vi "签名.vi"(10 "consumer secret":string, 11 "Signature Base string":string) -> (3 "Encoded Signature":string)   [LabVIEW 2016]
uses:
  <vilib>/LVH/i3 OAuth/Controls/Signature Method.ctl
  <vilib>/LVH/i3 External Encryption/labviewencryption/hash-types.ctl
  <vilib>/LVH/i3 External Encryption/i3-external-encryption.lvlib
  <vilib>/LVH/i3 OAuth/i3-oauth.lvlib
panel:
  out "长度":i32
  out "Base64 String":string
  in  "Signature Method":T1=enum."HMAC-SHA1"
  out "error out":errorcluster
  in  "error in (no error)":errorcluster
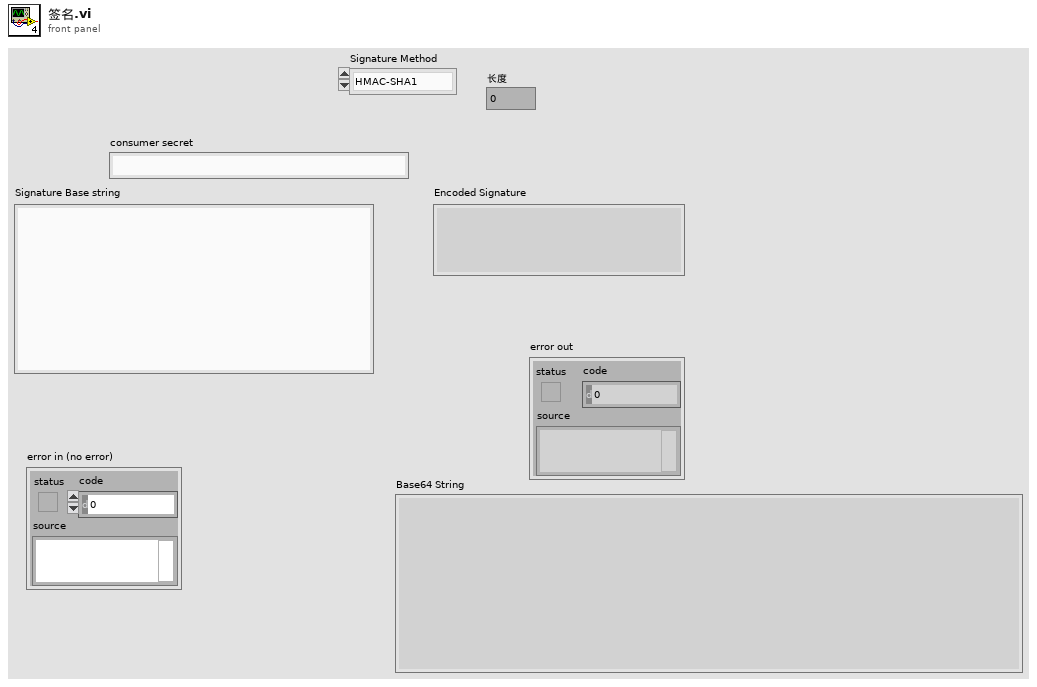
[diagram p1: front panel]
types:
  T1 = typedef "i3-oauth.lvlib/Signature Method.ctl" = enum16{"HMAC-MD5", "HMAC-SHA1", "HMAC-SHA224", "HMAC-SHA256", "HMAC-SHA384", "HMAC-SHA512"}
  T2 = typedef "i3-external-encryption.lvlib/hash-types.ctl" = enum16{"MD5", "SHA-1", "SHA-224", "SHA-256", "SHA-384", "SHA-512"}
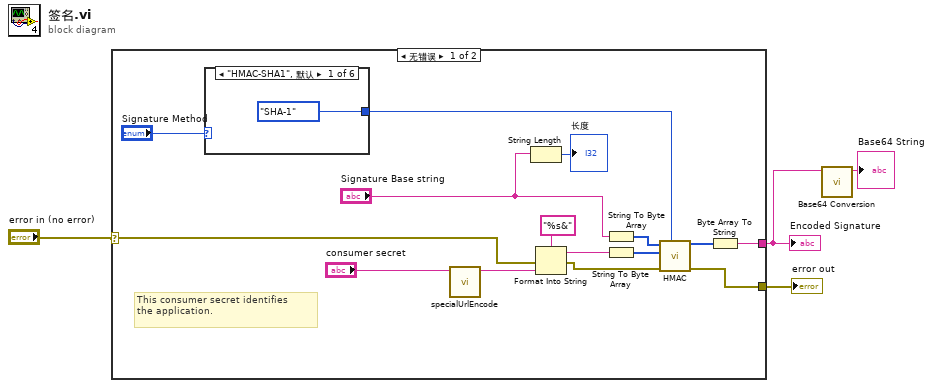
[diagram p0: block diagram]
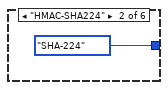
[diagram p2: hidden frame]
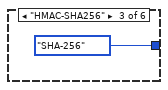
[diagram p3: hidden frame]
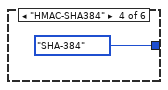
[diagram p4: hidden frame]
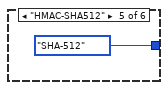
[diagram p5: hidden frame]
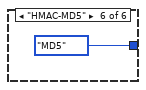
[diagram p6: hidden frame]
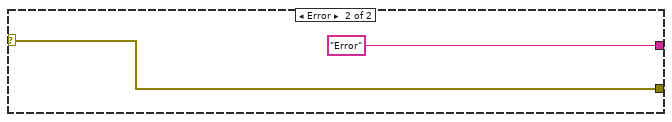
[diagram p7: hidden frame]
diagram:
  n1 = case shown="无错误" "error in (no error)" {
    selector: "error in (no error)" -> [w11 w27]
    tunnel: [w14 "Error"] -> w1
    tunnel: [w12 w27] -> w4
    frame No Error {
      # "This consumer secret identifies\nthe application."
      n2 = case shown="\"HMAC-SHA1\", 默认" "Signature Method" {
        tunnel: [hash-types."SHA-1" ("HASH-method 2") hash-types."SHA-224" ("HASH-method 2") hash-types."SHA-256" ("HASH-method 2") hash-types."SHA-384" ("HASH-method 2") hash-types."SHA-512" ("HASH-method 2") hash-types."MD5" ("HASH-method 2")] -> w10
        frame "HMAC-SHA1", Default {
        }
        frame "HMAC-SHA224" {
        }
        frame "HMAC-SHA256" {
        }
        frame "HMAC-SHA384" {
        }
        frame "HMAC-SHA512" {
        }
        frame "HMAC-MD5" {
        }
      }
      n3 = call "specialUrlEncode.vi"("str"="consumer secret") -> ("UrlEncode"=w7:string)  [unwired: 10 in]
      n4 = String Length(string="Signature Base string") -> (length=→"长度":i32)
      n5 = Format Into String(format string="%s&", error in=w11, w7) -> (resulting string=w15:string, error out=w13:errorcluster)  [unwired: 1 in]
      n6 = String To Byte Array(string="Signature Base string") -> (unsigned byte array=w18:u8[])
      n7 = String To Byte Array(string=w15) -> (unsigned byte array=w17:u8[])
      n8 = call <vilib>:"HMAC.vi"("HASH-method"=w10, "error in (no error)"=w13, "Key"=w17, "Message"=w18) -> ("error out"=w12:errorcluster, "HMAC digest"=w16:u8[])  [unwired: 5 in, 1 out]
      n9 = Byte Array To String(unsigned byte array=w16) -> (string=w14:string)
    }
    frame Error {
    }
  }
  "error out" <- w4
  "Encoded Signature" <- w1
  n10 = call <vilib>:"Base64 Conversion.vi"("String"=w1) -> ("Base64 String"=→"Base64 String":string)  [unwired: 10 in]
